vi "4D slow control.vi"(8 "Backward":bool, 9 "Forward":bool, 10 "Right":bool, 11 "Left":bool) -> (3 "Running Motor":bool)   [LabVIEW 2018]
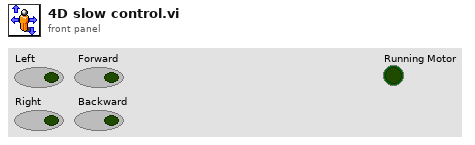
[diagram p1: front panel]
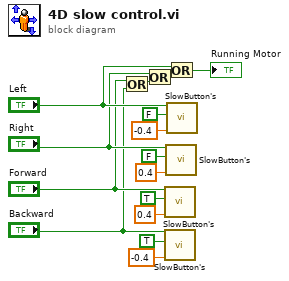
[diagram p0: block diagram]
diagram:
  n1 = Or(x="Forward", y="Backward") -> (x .or. y?=w7:bool)
  n2 = Or(x="Right", y=w7) -> (x .or. y?=w6:bool)
  n3 = call "SlowButton's.vi"("Speed"=0.4, "Straight"=TRUE, "Run"="Forward") -> ()  [unwired: 9 in]
  n4 = call "SlowButton's.vi"("Speed"=-0.4, "Straight"=TRUE, "Run"="Backward") -> ()  [unwired: 9 in]
  n5 = call "SlowButton's.vi"("Speed"=0.4, "Straight"=FALSE, "Run"="Right") -> ()  [unwired: 9 in]
  n6 = Or(x="Left", y=w6) -> (x .or. y?=→"Running Motor":bool)
  n7 = call "SlowButton's.vi"("Speed"=-0.4, "Straight"=FALSE, "Run"="Left") -> ()  [unwired: 9 in]
